vi "Force Sensors - L1-S1 model.vi"() -> ()   [LabVIEW 2019]
uses:
  <vilib>/Instr/_visa.llb/VISA Configure Serial Port (Instr).vi
  <vilib>/ptbypt/NI_PtbyPt.lvlib
panel:
  in  "coeff":dbl=0.0292
  out "Force in Newtons":dbl(graph)
  out "Sensor Raw Value":i32
  in  "COM Port-Sensor 1":refnum<visa-resource-name>="COM1"
  # "Sensor Calibration Values\n\nL1:          y = 0.4312 x ;    R-sq = 0.9998\n\nL2:          y = 0.7099 x ;    R-sq = 0.9961\n\nL3:          y = 0.5868 x ;    R-sq = 0.9951\n\nL4:          y = 0.5671 x ;    R-sq = 0.9982\n\nL5:          y = 0.5314 x ;    R-sq = 0.9968"
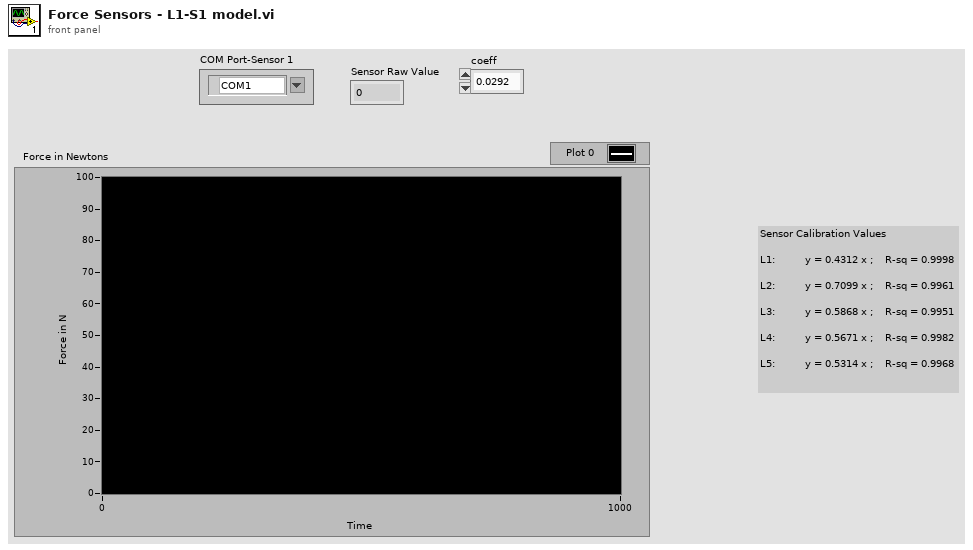
[diagram p1: front panel]
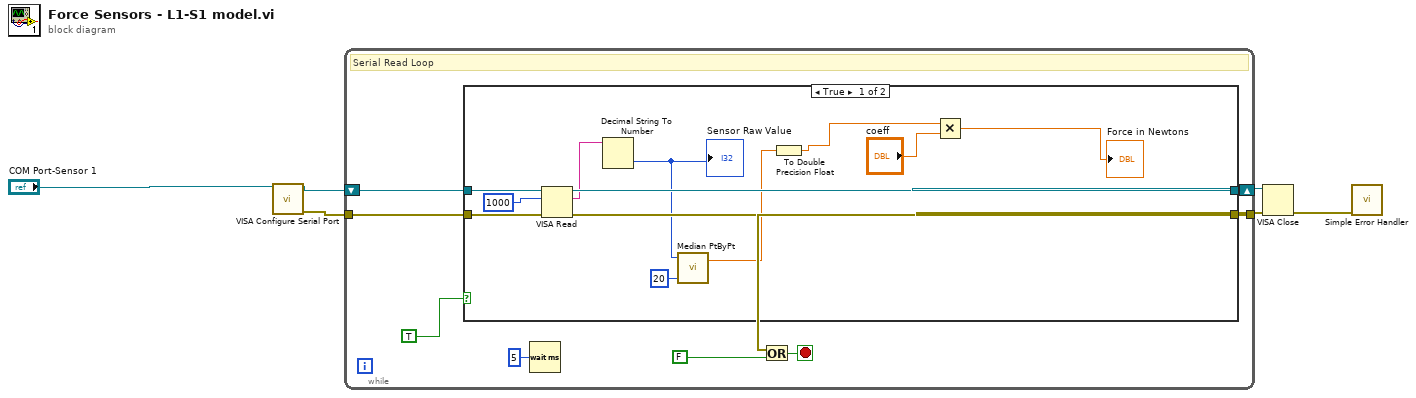
[diagram p0: block diagram]
diagram:
  n1 = call-poly "VISA Configure Serial Port"("VISA resource name"="COM Port-Sensor 1") -> ("VISA resource name out"=w2:refnum<visa-resource-name>, "error out"=w1:errorcluster)  [unwired: 9 in, 4 out]
  n2 = while {
    shift-right: [w14] -> w3
    shift-left: w2 -> [w10]
    tunnel: w1 -> [w9]
    tunnel: [w11] -> w4
    stop <- w12 stop-if-true
    # "Serial Read Loop"
    n3 = case shown="True" TRUE {
      tunnel: [w24 w28] -> w14
      tunnel: w10 -> [w26 w28]
      tunnel: [w23 w27] -> w11
      tunnel: w9 -> [w25 w27]
      frame True {
        n4 = VISA Read(VISA resource name=w26, byte count=u32 1000, error in (no error)=w25) -> (VISA resource name out=w24:refnum<visa-resource-name>, read buffer=w21:string, error out=w23:errorcluster)  [unwired: 1 out]
        n5 = Decimal String To Number(string=w21) -> (number=w20:i32)  [unwired: 2 in, 1 out]
        "Sensor Raw Value" <- w20
        n6 = call <vilib>:"Median PtByPt.vi"("sample length"=20, "x"=w20) -> ("median"=w18:dbl)  [unwired: 2 in, 1 out]
        n7 = To Double Precision Float(number=w18) -> (double precision float=w17:dbl)
        n8 = Multiply(x=w17, y="coeff") -> (x*y=→"Force in Newtons":dbl)
      }
      frame False {
      }
    }
    n9 = Wait (ms)(milliseconds to wait=u32 5) -> ()  [unwired: 1 out]
    n10 = Or(x=w11, y=FALSE) -> (x .or. y?=w12:bool)
  }
  n11 = VISA Close(VISA resource name=w3, error in (no error)=w4) -> (error out=w5:errorcluster)
  n12 = call <vilib>:"Simple Error Handler.vi"("error in (no error)"=w5) -> ()  [unwired: 1 in, 8 out]
